vi "DisplayGraph.vi"(9 "String":string, 11 "Waveform Graph":dbl[](graph)) -> ()   [LabVIEW 2012]
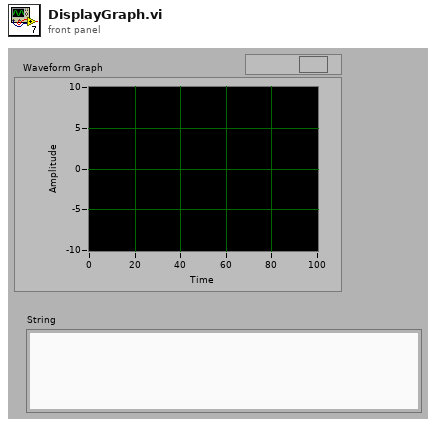
[diagram p1: front panel]
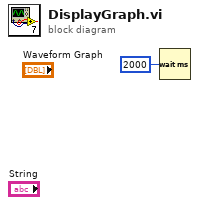
[diagram p0: block diagram]
diagram:
  n1 = Wait (ms)(milliseconds to wait=u32 2000) -> ()  [unwired: 1 out]
